vi "配置信息写入.vi"(10 "待保存数据":T2 {"曲线模型"."r^2" format="%.7g"}, 11 "模型选择":cluster{"参数":u8, "测量模式":u8, "量程":u8}) -> ()   [LabVIEW 2016, in "曲线模型.xctl"]
uses:
  <vilib>/Utility/config.llb/NI_LVConfig.lvlib
panel:
  # "标液浓度"
  # "F0"
  # "F1"
  # "吸光值显示"
  # "辅\n助\n计\n算\n区"
  # "样品一"
  # "样品二"
  # "样品三"
  # "样品四"
  # "样品五"
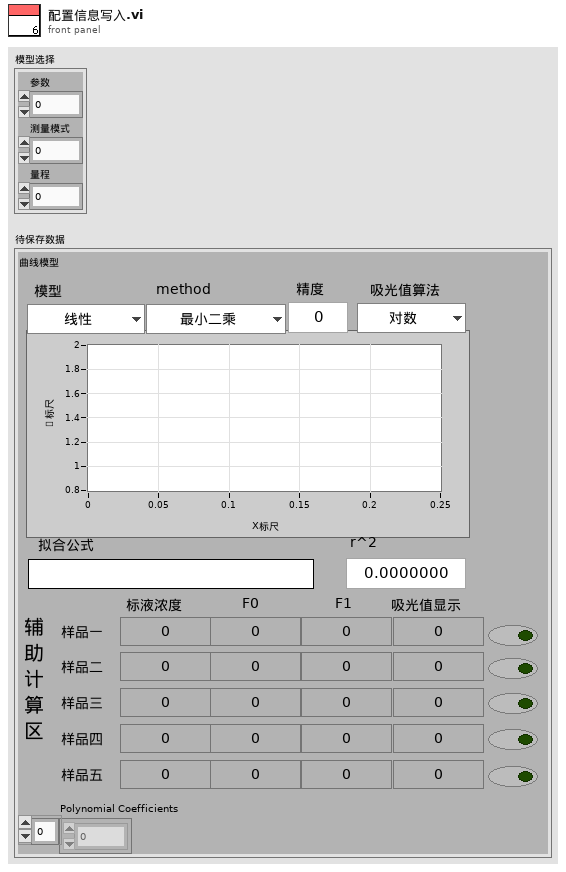
[diagram p1: front panel]
types:
  T1 = typedef "曲线模型.xctl/曲线模型外观.ctl" = cluster{"标液浓度1":dbl, "样品1 F0":dbl, "样品1 F1":dbl, "测量吸光度1":dbl, "样品1启用":bool, "标液浓度2":dbl, "样品2 F0":dbl, "样品2 F1":dbl, "测量吸光度2":dbl, "样品2启用":bool, "标液浓度3":dbl, "样品3 F0":dbl, "样品3 F1":dbl, "测量吸光度3":dbl, "样品3启用":bool, "标液浓度4":dbl, "样品4 F0":dbl, "样品4 F1":dbl, "测量吸光度4":dbl, "样品4启用":bool, "标液浓度5":dbl, "样品5 F0":dbl, "样品5 F1":dbl, "测量吸光度5":dbl, "样品5启用":bool, "模型":enum32{"线性", "多项式"}, "method":enum16{"最小二乘", "最小绝对残差", "Bisquare"}, "精度":dbl, "XY图":cluster{"X Values":dbl[], "Y Values":dbl[]}[], "拟合公式":string, "r^2":dbl, "吸光值算法":enum16{"对数", "减法"}}
  T2 = cluster{"曲线模型":T1, "Polynomial Coefficients":dbl[]}
  T3 = typedef "NI_LVConfig.lvlib/Config Data RefNum.ctl" = refnum<k1>
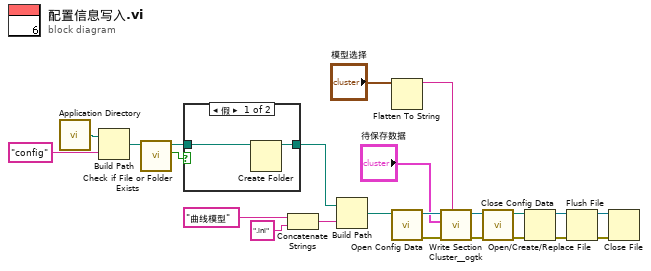
[diagram p0: block diagram]
diagram:
  n1 = call <vilib>:"Application Directory.vi"() -> ("Application Directory"=w7:path)
  n2 = Build Path(base path=w7, name or relative path="config" ("名称或相对路径")) -> (appended path=w6:path)
  n3 = call <vilib>:"Check if File or Folder Exists.vi"("path"=w6) -> ("file or folder exists?"=w4:bool, "dup path"=w5:path)  [unwired: 8 in, 1 out]
  n4 = case shown="假" w4 {
    tunnel: w5 -> [w25 w26]
    tunnel: [w24 w26] -> w3
    frame False {
      n5 = Create Folder(path (use dialog)=w25) -> (created path=w24:path)  [unwired: 2 in, 2 out]
    }
    frame True {
    }
  }
  n6 = Concatenate Strings("曲线模型" ("字符串"), ".ini" ("字符串")) -> (w10:string)
  n7 = Build Path(base path=w3, name or relative path=w10) -> (appended path=w17:path)
  n8 = Flatten To String(anything="模型选择") -> (data string=w9:string)  [unwired: 3 in, 2 out]
  n9 = call <vilib>:"Open Config Data.vi"("configuration file path"=w17) -> ("error out"=w14:errorcluster, "refnum"=w13:T3)  [unwired: 8 in, 1 out]
  n10 = call <userlib>:"Write Section Cluster__ogtk.vi"("section (optional)"=w9, "error in (no error)"=w14, "Section Formatted Cluster"="待保存数据", "refnum"=w13) -> ("error out"=w16:errorcluster, "dup refnum"=w15:T3)  [unwired: 6 in]
  n11 = call <vilib>:"Close Config Data.vi"("error in (no error)"=w16, "refnum"=w15) -> ("error out"=w19:errorcluster, "file path"=w18:path)  [unwired: 8 in]
  n12 = Open/Create/Replace File(file path (use dialog)=w18, error in=w19) -> (refnum out=w20:refnum<file>, error out=w22:errorcluster)  [unwired: 4 in, 1 out]
  n13 = Flush File(refnum=w20, error in=w22) -> (refnum out=w21:refnum<file>, error out=w23:errorcluster)
  n14 = Close File(refnum=w21, error in=w23) -> ()  [unwired: 2 out]
